vi "曲线取范围.vi"(9 "下限":dbl, 10 "上限":dbl, 11 "曲线In":cluster{"X":dbl[], "Y":dbl[]}[](array[cluster])) -> (3 "曲线Out":cluster{"X":dbl[], "Y":dbl[]}[](array[cluster]))   [LabVIEW 2020]
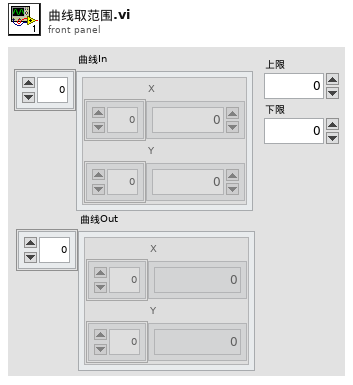
[diagram p1: front panel]
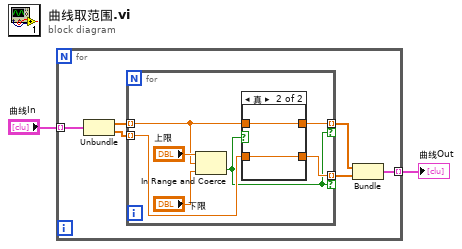
[diagram p0: block diagram]
diagram:
  n1 = for {
    tunnel: "曲线In" -> [w8] mode=indexing
    tunnel: [w3] -> w1 mode=indexing
    n2 = Unbundle(w8) -> ("X"=w7:dbl[], "Y"=w6:dbl[])
    n3 = for {
      tunnel: w7 -> [w13] mode=indexing
      tunnel: w6 -> [w12] mode=indexing
      tunnel: [w11] -> w5 mode=indexing if=w9
      tunnel: [w10] -> w4 mode=indexing if=w9
      n4 = In Range and Coerce(upper limit="上限", x=w13, lower limit="下限") -> (In Range?=w9:bool)  [unwired: 1 out]
      n5 = case shown="真" w9 {
        tunnel: w13 -> [_ w17]
        tunnel: w12 -> [_ w16]
        tunnel: [_ w17] -> w11
        tunnel: [_ w16] -> w10
        frame False {
        }
        frame True {
        }
      }
    }
    n6 = Bundle(w5, w4) -> (w3:cluster{dbl[], dbl[]})  [unwired: 1 in]
  }
  "曲线Out" <- w1
